vi "Root Path VIG.vi"(1 "Set Root VI's Path":path) -> (0 "Root VI's Path":path)   [LabVIEW 2018]
doc: "On first call, sets the Root VIs Path. This is meant to be done from the top level VI. Then on future calls, it reads that path as a basis for finding relative paths within the folder hierarchy from any VI on any target running either as source code or EXE, no matter how deep in the folder hierarchy they are on windows development system."
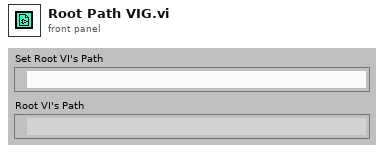
[diagram p1: front panel]
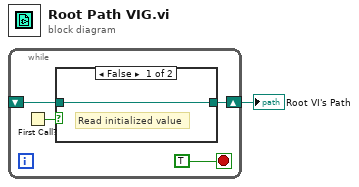
[diagram p0: block diagram]
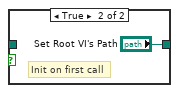
[diagram p2: hidden frame]
diagram:
  n1 = while {
    shift-right: [w3] -> w1
    shift-left: _ -> [w2]
    stop <- TRUE stop-if-true
    n2 = First Call?() -> (First Call?: T/F=w4:bool)
    n3 = case shown="False" w4 {
      tunnel: [w6 "Set Root VI's Path"] -> w3
      tunnel: w2 -> [w6 _]
      frame False {
        # "Read initialized value"
      }
      frame True {
        # "Init on first call"
      }
    }
  }
  "Root VI's Path" <- w1
